vi "GetCoeffsAndComp.vi"(8 "Apply Phase Correction?":bool=TRUE, 10 "mutedData":dbl[](array[numeric]), 11 "TubingCorrectionFile":path) -> (1 "boostedDataNaNdEnds":dbl[](array[numeric]), 2 "boostedData":dbl[](array[numeric]))   [LabVIEW 2016]
uses:
  Globals/Meas_global.vi
panel:
  in  "Refresh Button":bool
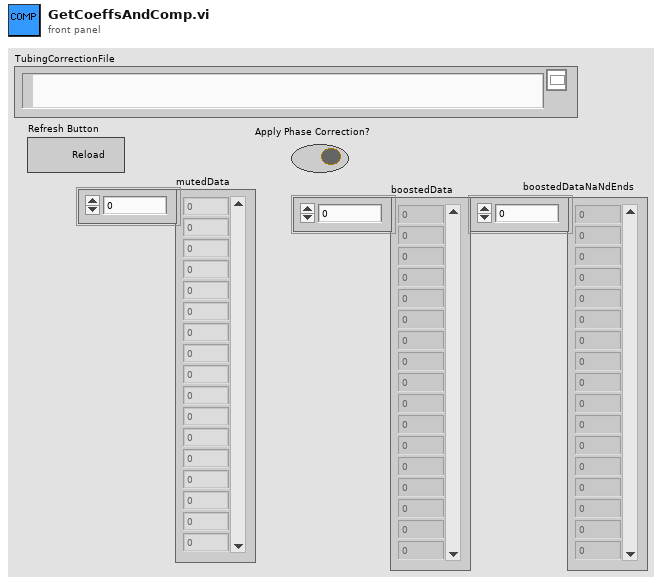
[diagram p1: front panel]
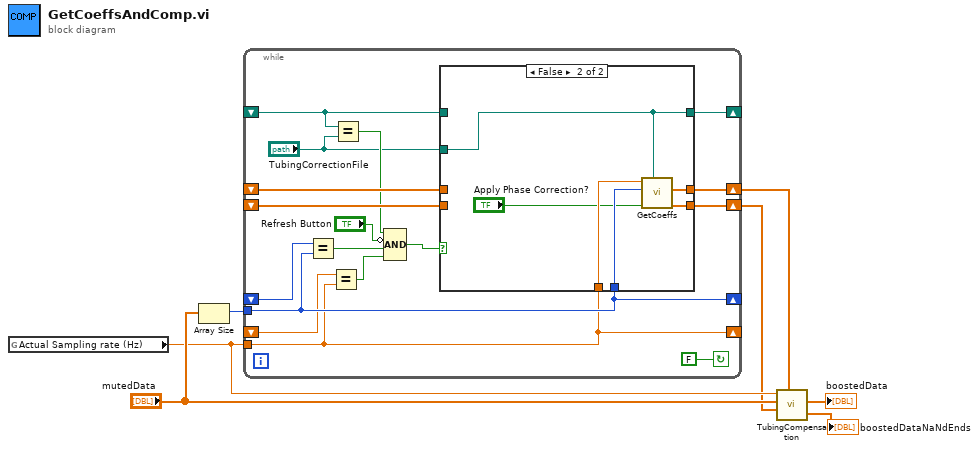
[diagram p0: block diagram]
diagram:
  n1 = global read "Meas_global.vi" "Actual Sampling rate (Hz)"() -> (w4:dbl)
  n2 = Array Size(array="mutedData") -> (size(s)=w6:i32)
  n3 = while {
    shift-right: [w23] -> w3
    shift-left: _ -> [w24]
    shift-right: [w20] -> _
    shift-left: _ -> [w21]
    shift-right: [w18] -> _
    shift-left: _ -> [w19]
    tunnel: w6 -> [w20]
    tunnel: w4 -> [w18]
    shift-right: [w15] -> _
    shift-left: _ -> [w8]
    shift-right: [w14] -> w2
    shift-left: _ -> [w13]
    stop <- FALSE continue-if-true
    n4 = Equal?(x=w21, y=w20) -> (x = y?=w16:bool)
    n5 = Equal?(x=w19, y=w18) -> (x = y?=w17:bool)
    n6 = Equal?(x=w8, y="TubingCorrectionFile") -> (x = y?=w10:bool)
    n7 = Compound Arithmetic op=AND(w10, invert "Refresh Button", w16, w17) -> (w12:bool)
    n8 = case shown="False" w12 {
      tunnel: [w27 w33] -> w23
      tunnel: w24 -> [w27 _]
      tunnel: w18 -> [_ w32]
      tunnel: w20 -> [_ w31]
      tunnel: [w26 w28] -> w15
      tunnel: w8 -> [w26 _]
      tunnel: [w25 w29] -> w14
      tunnel: w13 -> [w25 _]
      tunnel: "TubingCorrectionFile" -> [_ w28]
      frame True {
      }
      frame False {
        n9 = call "GetCoeffs.vi"("PathToFile"=w28, "Apply Phase Correction?"="Apply Phase Correction?", "SignalLength"=w31, "fs (Hz)"=w32) -> ("NyquistLimitedPhase"=w29:dbl[], "NyquistLimitedCoefficients"=w33:dbl[])  [unwired: 6 in]
      }
    }
  }
  n10 = call "TubingCompensation.vi"("NyquistLimitedCoefficients"=w3, "NyquistLimitedPhase"=w2, "mutedData"="mutedData", "SamplingFreq"=w4) -> ("boostedDataNaNdEnds"=→"boostedDataNaNdEnds":dbl[], "boostedData"=→"boostedData":dbl[])  [unwired: 6 in]
